vi "TS_RST_MODE - Type.vi"(8 "error in (no error)":errorcluster) -> (0 "error out":errorcluster, 3 "TS_RST_MODE_VALUE":i32)   [LabVIEW 2015]
doc: "<b>Buffer policy settings can be only unsafe in xiAPI LabVIEW library</b>\nUNSAFE : User gets pointer to internally allocated circle buffer and data may be overwritten by device.\nSAFE : Data from device will be copied to user allocated buffer or xiApi allocated memory."
uses:
  C:/GIT/Cameras3.x/Integrations/Labview/xiLib/xiLIB_32bit/xiLIB/xiCamLib/API/x86/xiApi.NET.dll
  xiLIB_32bit/xiLIB/xiCamLib/API/x86/xiApi.NET.dll
  TS_RST_MODE.ctl
panel:
  in  "TS_RST_MODE":T1
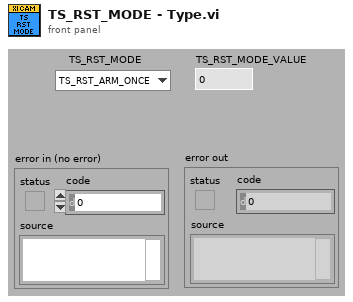
[diagram p1: front panel]
types:
  T1 = typedef "TS_RST_MODE.ctl" = enum16{"TS_RST_ARM_ONCE", "TS_RST_ARM_PERSIST"}
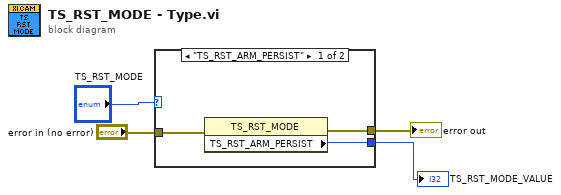
[diagram p0: block diagram]
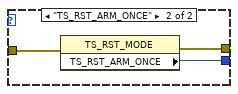
[diagram p2: hidden frame]
diagram:
  n1 = case shown="\"TS_RST_ARM_PERSIST\"" "TS_RST_MODE" {
    tunnel: "error in (no error)" -> [w7 w10]
    tunnel: [w6 w9] -> w3
    tunnel: [w5 w8] -> w2
    frame "TS_RST_ARM_PERSIST" {
      n2 = property class="TS_RST_MODE"(error in=w7) -> (error out=w6:errorcluster, "TS_RST_ARM_PERSIST"=w5:i32)  [unwired: 1 in, 1 out]
    }
    frame "TS_RST_ARM_ONCE" {
      n3 = property class="TS_RST_MODE"(error in=w10) -> (error out=w9:errorcluster, "TS_RST_ARM_ONCE"=w8:i32)  [unwired: 1 in, 1 out]
    }
  }
  "error out" <- w3
  "TS_RST_MODE_VALUE" <- w2
